vi "Obtain Broadcast Events for Registration.vi"(8 "error in":errorcluster) -> (0 "error out":errorcluster, 2 "Already running?":bool, 3 "FT-818 CW Key Control Broadcast Events":T1)   [LabVIEW 2026, in "FT-818 CW Key Control.lvlib"]
doc: "Return the broadcast event refnums so the module's caller can register for the module's broadcast events.\n_____\nBased on DQMH Dev Tools: Project Template 7.1.2.1547."
uses:
  FT-818 CW Key Control.lvlib
  Broadcast Events--cluster.ctl
  Did Init Argument--cluster.ctl
  Status Updated Argument--cluster.ctl
  Error Reported Argument--cluster.ctl
  Stop Argument--cluster.ctl
  Get Module Execution Status Argument--cluster.ctl
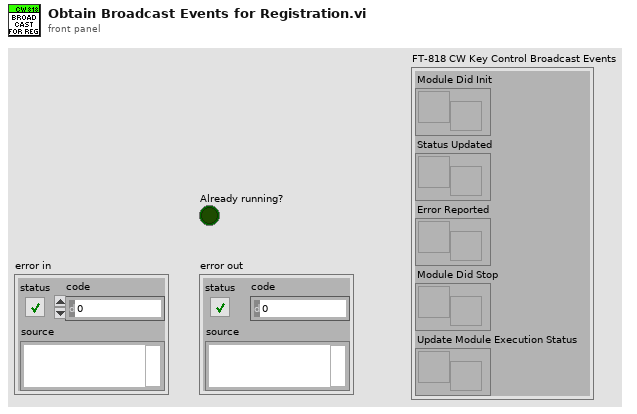
[diagram p1: front panel]
types:
  T1 = typedef "FT-818 CW Key Control.lvlib/Broadcast Events--cluster.ctl" = cluster{"Module Did Init":refnum<user-event>, "Status Updated":refnum<user-event>, "Error Reported":refnum<user-event>, "Module Did Stop":refnum<user-event>, "Update Module Execution Status":refnum<user-event>}
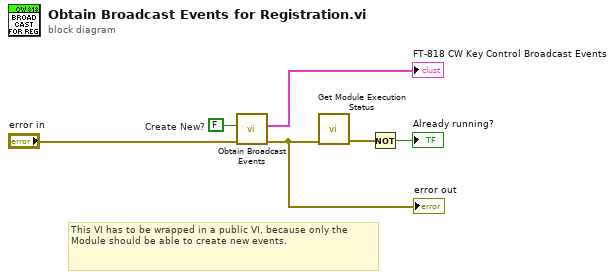
[diagram p0: block diagram]
diagram:
  w5 = FALSE  # Create New?
  # "This VI has to be wrapped in a public VI, because only the Module should be able to create new events."
  n1 = call "Obtain Broadcast Events.vi"("error in"="error in", "Create New? (F)"=w5) -> ("error out"=w4:errorcluster, "FT-818 CW Key Control Broadcast Events"=→"FT-818 CW Key Control Broadcast Events":T1)  [unwired: 8 in]
  "error out" <- w4
  n2 = call "Get Module Execution Status.vi"("error in"=w4) -> ("error out"=w3:errorcluster)  [unwired: 10 in]
  n3 = Not(x=w3) -> (.not. x?=→"Already running?":bool)
